vi "SubVHist.vi"(9 "Mouse in":T2, 10 "T":dbl, 11 "image data":T1) -> (1 "24-bit pixmap":u32[][](array[numeric]), 2 "new picture":picture, 3 "Mouse out":T2)   [LabVIEW 2020]
uses:
  <vilib>/Utility/miscctls.llb/LVMouseTypeDef.ctl
  <vilib>/picture/picture.llb/imagedata.ctl
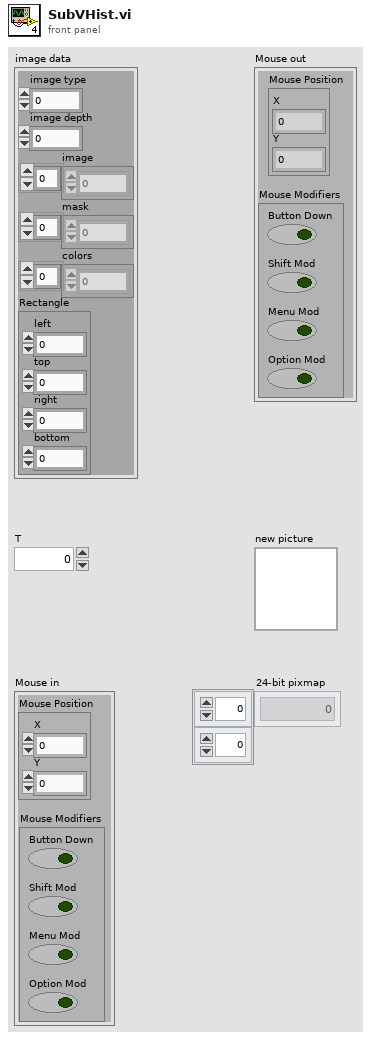
[diagram p1: front panel]
types:
  T1 = typedef "imagedata.ctl" = cluster{"image type":i32, "image depth":i32, "image":u8[], "mask":u8[], "colors":u32[], "Rectangle":cluster{"left":i16, "top":i16, "right":i16, "bottom":i16}}
  T2 = typedef "LVMouseTypeDef.ctl" = cluster{"Mouse Position":cluster{"X":i32, "Y":i32}, "Mouse Modifiers":cluster{"Button Down":bool, "Shift Mod":bool, "Menu Mod":bool, "Option Mod":bool}}
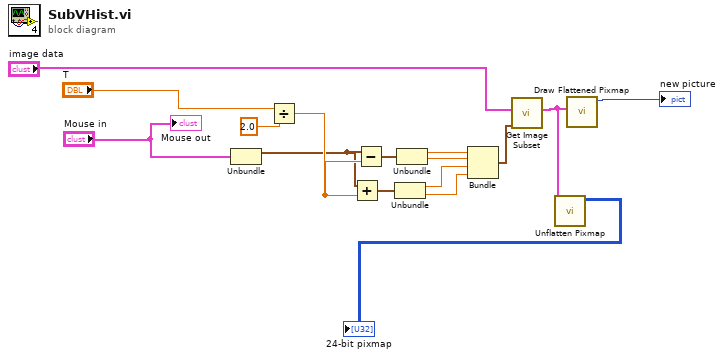
[diagram p0: block diagram]
diagram:
  n1 = Unbundle("Mouse in") -> ("Mouse Position"=w5:cluster{"X":i32, "Y":i32})  [unwired: 1 out]
  n2 = Divide(x="T", y=2.0) -> (x/y=w8:dbl)
  n3 = Add(x=w5, y=w8) -> (x+y=w7:cluster{"X":dbl, "Y":dbl})
  n4 = Subtract(x=w5, y=w8) -> (x-y=w6:cluster{"X":dbl, "Y":dbl})
  n5 = Unbundle(w7) -> ("X"=w11:dbl, "Y"=w12:dbl)
  n6 = Unbundle(w6) -> ("X"=w9:dbl, "Y"=w10:dbl)
  n7 = Bundle("X"=w9, "Y"=w10, "X"=w11, "Y"=w12) -> (w13:cluster{"X":dbl, "Y":dbl, "X":dbl, "Y":dbl})  [unwired: 1 in]
  n8 = call <vilib>:"Get Image Subset.vi"("subset rect"=w13, "image data"="image data") -> ("image subset"=w15:T1)  [unwired: 4 in, 1 out]
  n9 = call <vilib>:"Unflatten Pixmap.vi"("image data"=w15) -> ("24-bit pixmap"=→"24-bit pixmap":u32[][])  [unwired: 4 in, 6 out]
  n10 = call <vilib>:"Draw Flattened Pixmap.vi"("image data"=w15) -> ("new picture"=→"new picture":picture)  [unwired: 8 in]
  "Mouse out" <- "Mouse in"
